vi "PMC_DEMO.vi"() -> ()   [LabVIEW 2010]
panel:
  out "Connect":bool
  in  "mon":bool
  in  "?":bool
  in  "?":bool
  in  "AXIS":u16(ring)=2 items=["X", "Y", "X,Y"]
  in  "AXIS":u16(ring)=2 items=["X", "Y", "X,Y"]
  in  "STOP HOME":bool
  in  "AXIS":u16(ring) items=["X", "Y", "X&Y"]
  in  "AXIS":u16(ring) items=["X", "Y", "X&Y"]
  in  "HOME":bool
  in  "STOP":bool
  in  "AXIS":u16(ring) items=["X", "Y", "XY"]
  in  "Y Position(ABS)":dbl=1000.0 format="%#_8g"
  in  "X Position(ABS)":dbl=2000.0 format="%#_8g"
  in  "MOVE(ABS)":bool
  in  "MOVE(REL)":bool
  in  "X Position(REL)":dbl=1000.0 format="%#_8g"
  in  "Y Position(REL)":dbl=2000.0 format="%#_8g"
  out "MON":bool
  out "RUN (Y)":bool
  out "HOMing(Y)":bool
  out "Limit- (Y)":bool=TRUE
  out "Limit+ (Y)":bool=TRUE
  out "InPOS (Y)":bool=TRUE
  out "RUN  (X)":bool
  out "HOMing  (X)":bool
  out "Limit-  (X)":bool
  out "Limit+  (X)":bool
  out "InPOS (X)":bool=TRUE
  out "Speed(Y)":i32
  out "Speed(X)":i32
  out "Position(Y)":i32
  out "Position(X)":i32
  in  "Drive speed Set":bool
  out "Spped":u32=1000
  in  "Axis":u16(ring) items=["X", "Y"]
  in  "Drive Speed Number":u16(ring) items=["Drive Speed 1", "Drive Speed 2", "Drive Speed 3", "Drive Speed 4"]
  in  "SPEED(1~4)":string="4"
  in  "AXIS":u16(ring) items=["X", "Y"]
  in  "Speed Set":bool
  in  "BAUD(9600)":string="9600"
  in  "SET COM":bool
  out "Version":string
  in  "baud rate (9600)":u32=9600 caption="보 전송속도(9600)"
  in  "Port":refnum<visa-resource-name>="COM4" caption="VISA 리소스 이름"
  in  "SET":bool
  in  "EXIT":bool
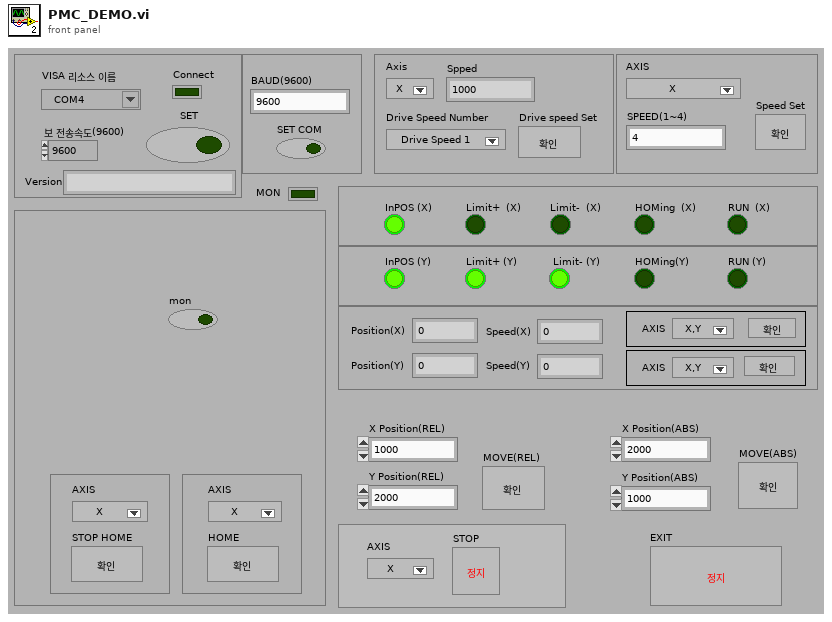
[diagram p1: front panel]
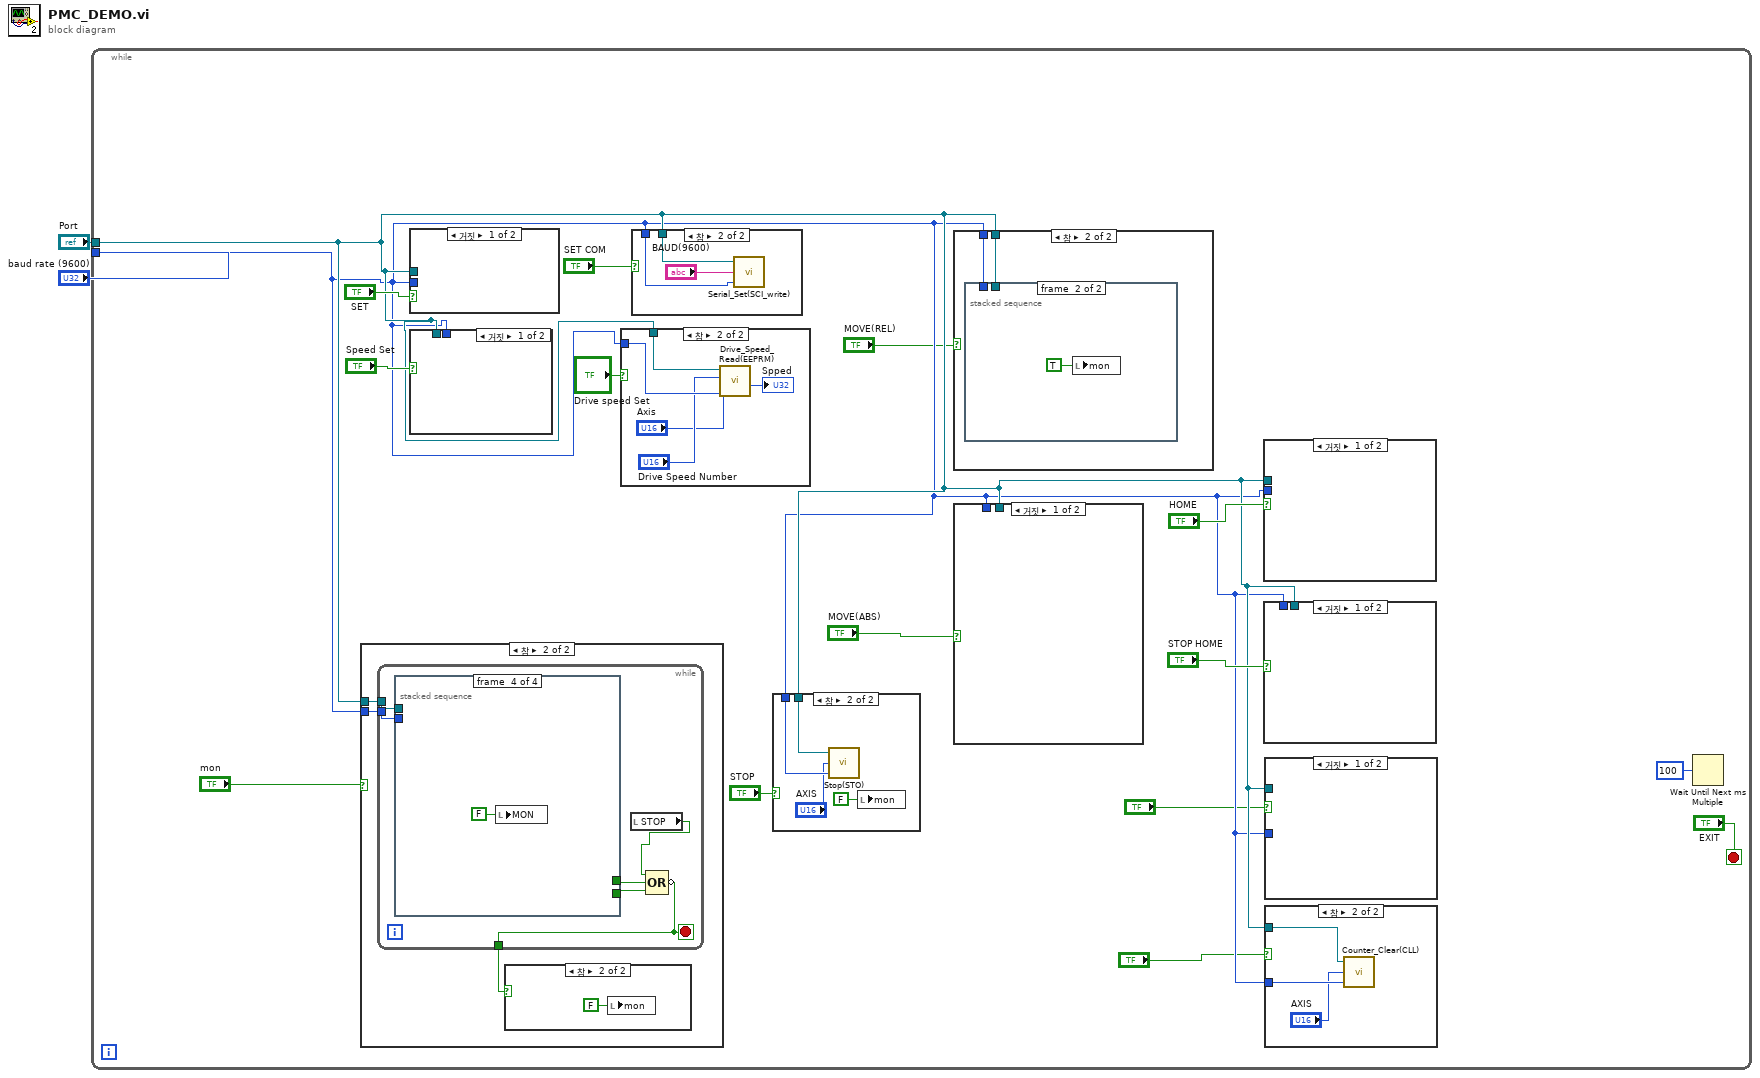
[diagram p0: block diagram]
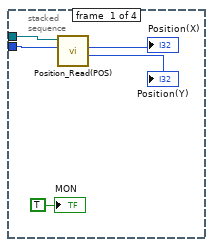
[diagram p4: hidden frame]
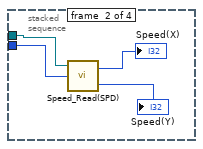
[diagram p5: hidden frame]
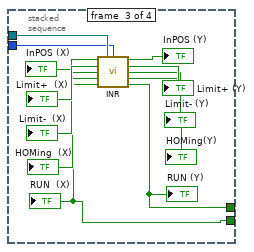
[diagram p6: hidden frame]
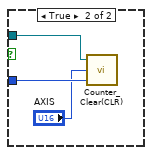
[diagram p8: hidden frame]
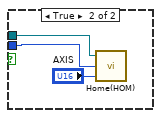
[diagram p9: hidden frame]
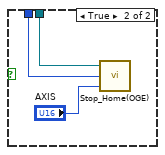
[diagram p10: hidden frame]
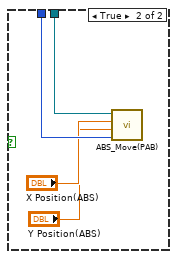
[diagram p12: hidden frame]
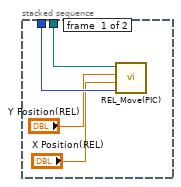
[diagram p14: hidden frame]
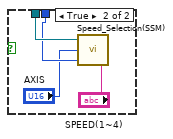
[diagram p16: hidden frame]
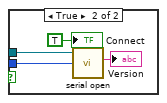
[diagram p18: hidden frame]
diagram:
  n1 = while {
    tunnel: "Port" -> [w8]
    tunnel: "baud rate (9600)" -> [w7]
    stop <- "EXIT" stop-if-true
    n2 = case shown="참" "mon" {
      tunnel: w8 -> [_ w21]
      tunnel: w7 -> [_ w20]
      frame False {
      }
      frame True {
        n3 = while {
          tunnel: w21 -> [w28]
          tunnel: w20 -> [w27]
          tunnel: [w24] -> w19
          stop <- w24 stop-if-true
          n4 = stacked-sequence {
            tunnel: w28 -> [w33 w37 w49 _]
            tunnel: w27 -> [w32 w36 w48 _]
            tunnel: [_ _ w39 _] -> w26
            tunnel: [_ _ w38 _] -> w25
            frame #0 {
              n5 = call <userlib>:"Position_Read(POS).vi"("baud rate (9600)"=w32, "Port"=w33) -> ("Position(Y)"=→"Position(Y)":i32, "Position(X)"=→"Position(X)":i32)  [unwired: 2 in, 3 out]
              "MON" <- TRUE ("MON")
            }
            frame #1 {
              n6 = call <userlib>:"Speed_Read(SPD).vi"("baud rate (9600)"=w36, "Port"=w37) -> ("Speed(Y)"=→"Speed(Y)":i32, "Speed(X)"=→"Speed(X)":i32)  [unwired: 1 in, 1 out]
            }
            frame #2 {
              n7 = call <userlib>:"INR.vi"("Port"=w49, "baud rate (9600)"=w48) -> ("InPOS (X)"=→"InPOS (X)":bool, "InPOS (Y)"=→"InPOS (Y)":bool, "Limit+  (X)"=→"Limit+  (X)":bool, "Limit+ (Y)"=→"Limit+ (Y)":bool, "Limit-  (X)"=→"Limit-  (X)":bool, "Limit- (Y)"=→"Limit- (Y)":bool, "HOMing  (X)"=→"HOMing  (X)":bool, "HOMing(Y)"=→"HOMing(Y)":bool, "RUN  (X)"=w39:bool, "RUN (Y)"=w38:bool)  [unwired: 4 out]
              "RUN  (X)" <- w39
              "RUN (Y)" <- w38
            }
            frame #3 {
              n8 = local write "MON"(FALSE ("MON")) -> ()
            }
          }
          n9 = local read "STOP"() -> (w23:bool)
          n10 = Compound Arithmetic op=OR(w23, w25, w26) -> (invert w24:bool)
        }
        n11 = case shown="참" w19 {
          frame False {
          }
          frame True {
            n12 = local write "mon"(FALSE ("mon")) -> ()
          }
        }
      }
    }
    n13 = case shown="거짓" "SET" {
      tunnel: w8 -> [_ w93]
      tunnel: w7 -> [_ w92]
      frame False {
      }
      frame True {
        n14 = call <userlib>:"serial open.vi"("baud rate (9600)"=w92, "Port"=w93) -> ("Version"=→"Version":string)  [unwired: 2 in, 2 out]
        "Connect" <- TRUE ("Connect")
      }
    }
    n15 = case shown="거짓" "Speed Set" {
      tunnel: w8 -> [_ w86]
      tunnel: w7 -> [_ w85]
      frame False {
      }
      frame True {
        n16 = call <userlib>:"Speed_Selection(SSM).vi"("SPEED(1~4)"="SPEED(1~4)", "baud rate (9600)"=w85, "AXIS"="AXIS", "Port"=w86) -> ()  [unwired: 2 out]
      }
    }
    n17 = case shown="참" "Drive speed Set" {
      tunnel: w8 -> [_ w82]
      tunnel: w7 -> [_ w81]
      frame False {
      }
      frame True {
        n18 = call <userlib>:"Drive_Speed_Read(EEPRM).vi"("baud rate (9600)"=w81, "Axis"="Axis", "Drive Speed Number"="Drive Speed Number", "Port"=w82) -> ("Spped"=→"Spped":u32)  [unwired: 1 in, 3 out]
      }
    }
    n19 = case shown="참" "SET COM" {
      tunnel: w8 -> [_ w89]
      tunnel: w7 -> [_ w87]
      frame False {
      }
      frame True {
        n20 = call <userlib>:"Serial_Set(SCI_write).vi"("baud rate (9600)"=w87, "BAUD(9600)"="BAUD(9600)", "Port"=w89) -> ()  [unwired: 2 out]
      }
    }
    n21 = case shown="참" "STOP" {
      tunnel: w8 -> [_ w66]
      tunnel: w7 -> [_ w65]
      frame False {
      }
      frame True {
        n22 = call <userlib>:"Stop(STO).vi"("baud rate (9600)"=w65, "AXIS"="AXIS", "Port"=w66) -> ()  [unwired: 2 out]
        n23 = local write "mon"(FALSE ("mon")) -> ()
      }
    }
    n24 = case shown="참" "MOVE(REL)" {
      tunnel: w8 -> [_ w72]
      tunnel: w7 -> [_ w71]
      frame False {
      }
      frame True {
        n25 = stacked-sequence {
          tunnel: w72 -> [w76 _]
          tunnel: w71 -> [w75 _]
          frame #0 {
            n26 = call <userlib>:"REL_Move(PIC).vi"("baud rate (9600)"=w75, "X Position(REL)"="X Position(REL)", "Y Position(REL)"="Y Position(REL)", "Port"=w76) -> ()  [unwired: 1 in, 2 out]
          }
          frame #1 {
            n27 = local write "mon"(TRUE ("MON")) -> ()
          }
        }
      }
    }
    n28 = case shown="거짓" "MOVE(ABS)" {
      tunnel: w8 -> [_ w70]
      tunnel: w7 -> [_ w69]
      frame False {
      }
      frame True {
        n29 = call <userlib>:"ABS_Move(PAB).vi"("baud rate (9600)"=w69, "Y Position(ABS)"="Y Position(ABS)", "X Position(ABS)"="X Position(ABS)", "Port"=w70) -> ()  [unwired: 2 in, 3 out]
      }
    }
    n30 = case shown="거짓" "HOME" {
      tunnel: w8 -> [_ w59]
      tunnel: w7 -> [_ w58]
      frame False {
      }
      frame True {
        n31 = call <userlib>:"Home(HOM).vi"("AXIS"="AXIS", "baud rate (9600)"=w58, "Port"=w59) -> ()  [unwired: 2 out]
      }
    }
    n32 = case shown="거짓" "STOP HOME" {
      tunnel: w8 -> [_ w62]
      tunnel: w7 -> [_ w61]
      frame False {
      }
      frame True {
        n33 = call <userlib>:"Stop_Home(OGE).vi"("AXIS"="AXIS", "baud rate (9600)"=w61, "Port"=w62) -> ()  [unwired: 2 out]
      }
    }
    n34 = case shown="거짓" "?" {
      tunnel: w8 -> [_ w56]
      tunnel: w7 -> [_ w55]
      frame False {
      }
      frame True {
        n35 = call <userlib>:"Counter_Clear(CLR).vi"("baud rate (9600)"=w55, "AXIS"="AXIS", "Port"=w56) -> ()  [unwired: 2 out]
      }
    }
    n36 = case shown="참" "?" {
      tunnel: w8 -> [_ w53]
      tunnel: w7 -> [_ w52]
      frame False {
      }
      frame True {
        n37 = call <userlib>:"Counter_Clear(CLL).vi"("baud rate (9600)"=w52, "AXIS"="AXIS", "Port"=w53) -> ()  [unwired: 2 out]
      }
    }
    n38 = Wait Until Next ms Multiple(millisecond multiple=u32 100 ("ms 배수")) -> ()  [unwired: 1 out]
  }
